vi "Write password.vi"(8 "error in (no error)":errorcluster, 10 "password":string, 11 "protection settings in":refnum<class "protection settings.lvclass">) -> (0 "error out":errorcluster, 3 "protection settings out":refnum<class "protection settings.lvclass">)   [LabVIEW 2013, in "protection settings.lvclass"]
uses:
  protection settings.lvclass
  protection settings.lvclass/protection settings.ctl
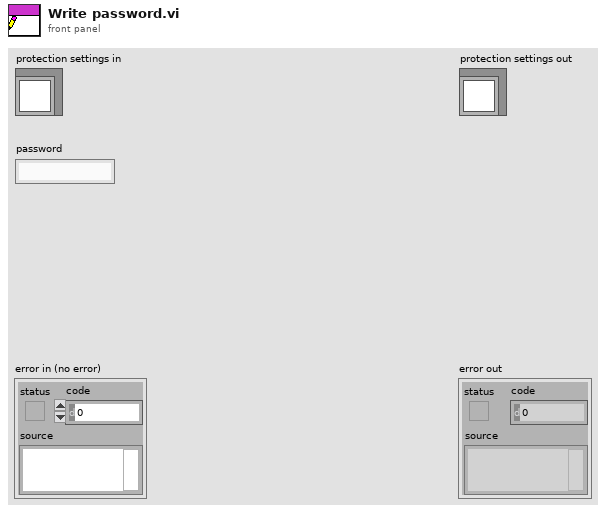
[diagram p1: front panel]
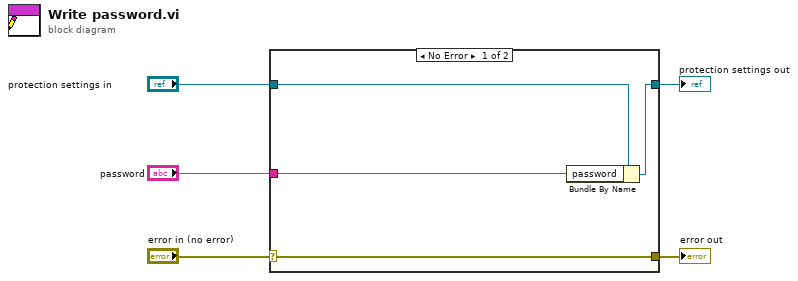
[diagram p0: block diagram]
diagram:
  n1 = case shown="No Error" "error in (no error)" {
    selector: "error in (no error)" -> [w9 w10]
    tunnel: [w9 w10] -> w4
    tunnel: [w7 w11] -> w2
    tunnel: "protection settings in" -> [w8 w11]
    tunnel: "password" -> [w6 _]
    frame No Error {
      n2 = Bundle By Name(cluster=w8, "password"=w6) -> (w7:refnum<class "protection settings.lvclass">)
    }
    frame Error {
    }
  }
  "error out" <- w4
  "protection settings out" <- w2
